vi "全局 环境参数.vi"() -> ()   [LabVIEW 2016, in "数据传输系统-02.lvlib"]
panel:
  out "columns输出":string[](array[string])
  in  "环境参数":string[][](array[string])
  # "时间"
  # "电压"
  # "温度"
  # "湿度"
  # "GPS经度"
  # "GPS纬度"
  # "BDS纬度"
  # "BDS纬度"
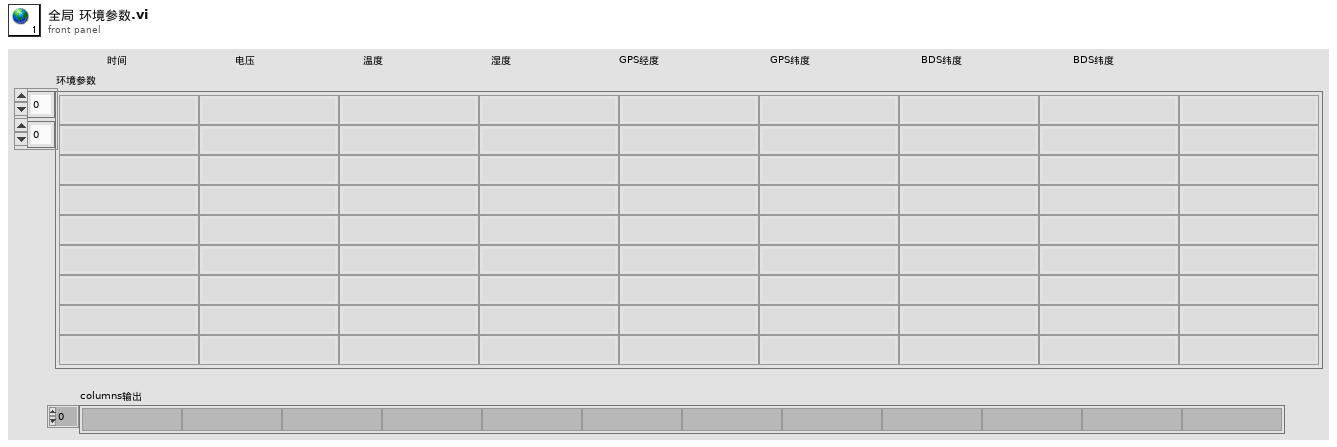
[diagram p1: front panel]
diagram:
